vi "Read timeToBlindSpotExit_min.vi"(8 "error in (no error)":errorcluster, 11 "Zenith in":refnum<class "Zenith.lvclass">) -> (0 "error out":errorcluster, 2 "timeToBlindSpotExit_min":dbl[unit], 3 "Zenith out":refnum<class "Zenith.lvclass">)   [LabVIEW 2014, in "TCSDataDefinitions.lvlib" / "TCSPublicStatus.lvlib" / "Limits.lvlib" / "Zenith.lvclass"]
uses:
  Zenith.lvclass
  Zenith.lvclass/Zenith.ctl
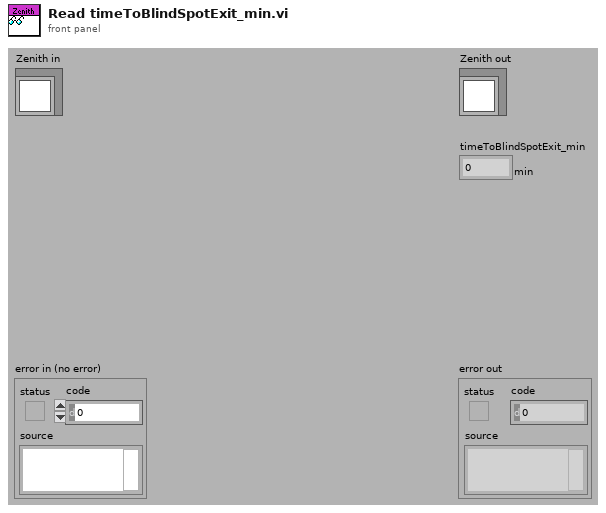
[diagram p1: front panel]
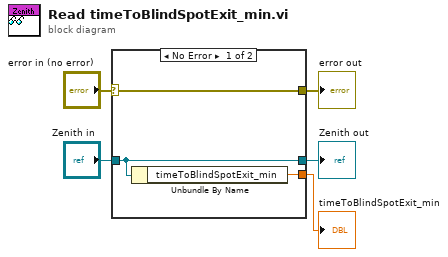
[diagram p0: block diagram]
diagram:
  n1 = case shown="No Error" "error in (no error)" {
    selector: "error in (no error)" -> [w8 w9]
    tunnel: [w8 w9] -> w4
    tunnel: [w7 w10] -> w2
    tunnel: "Zenith in" -> [w7 w10]
    tunnel: [w6 _] -> w1
    frame No Error {
      n2 = Unbundle By Name(w7) -> ("timeToBlindSpotExit_min"=w6:dbl[unit])
    }
    frame Error {
    }
  }
  "error out" <- w4
  "Zenith out" <- w2
  "timeToBlindSpotExit_min" <- w1
